vi "SendClusterClientSide.vi"() -> ()   [LabVIEW 2019]
panel:
  in  "Stop From Client Side":bool
  out "error out":errorcluster
  out "Side":string
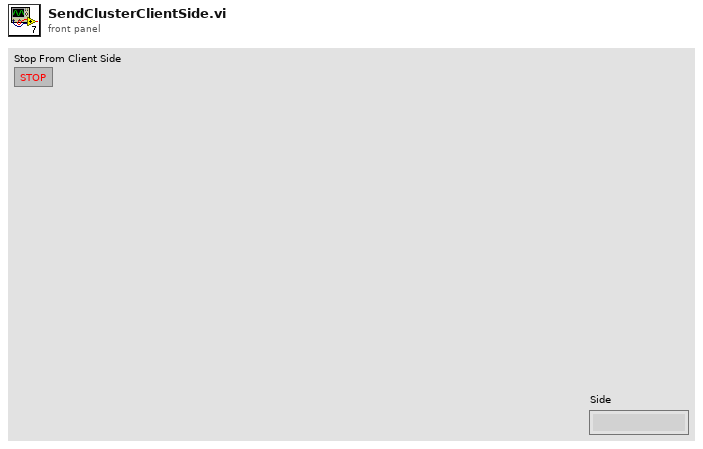
[diagram p1: front panel]
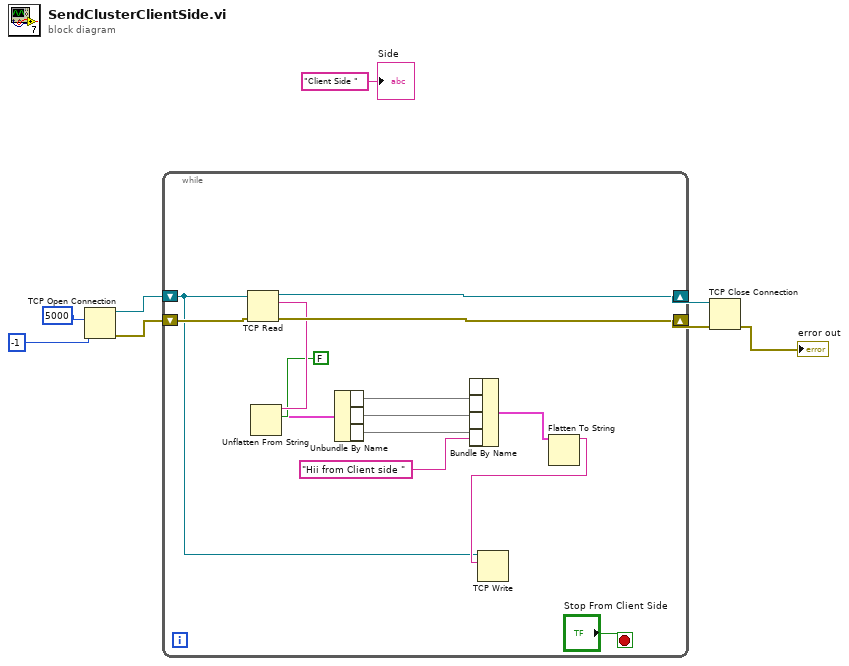
[diagram p0: block diagram]
diagram:
  n1 = TCP Open Connection(remote port or service name=u16 5000, timeout ms (60000)=-1) -> (connection ID=w1:refnum<k5>, error out=w4:errorcluster)  [unwired: 3 in]
  n2 = while {
    shift-right: [w20] -> w3
    shift-left: w4 -> [w21]
    shift-right: [w22] -> w5
    shift-left: w1 -> [w10]
    stop <- "Stop From Client Side" stop-if-true
    n3 = TCP Read(connection ID=w10, error in (no error)=w21) -> (connection ID out=w22:refnum<k5>, data out=w19:string, error out=w20:errorcluster)  [unwired: 3 in]
    n4 = Unflatten From String(binary string=w19, data includes array or string size? (T)=FALSE) -> (value=w17:cluster{})  [unwired: 3 in, 2 out]
    n5 = Unbundle By Name "Unbundle By Name"(w17) -> (w16, w15, w14)
    n6 = Bundle By Name(w16, w15, w14, "Hii from Client side ") -> (w12:cluster{})  [unwired: 1 in]
    n7 = Flatten To String(anything=w12) -> (data string=w11:string)  [unwired: 3 in, 2 out]
    n8 = TCP Write(connection ID=w10, data in=w11) -> ()  [unwired: 2 in, 3 out]
  }
  n9 = TCP Close Connection(connection ID=w5, error in (no error)=w3) -> (error out=→"error out":errorcluster)  [unwired: 1 in, 1 out]
  "Side" <- "Client Side " ("Side")
